vi "Send.vi"(8 "error in":errorcluster, 11 "Expedited Download Transfer in":refnum<class "Segmented Download Transfer.lvclass">) -> (0 "error out":errorcluster, 3 "Expedited Download Transfer out":refnum<class "Segmented Download Transfer.lvclass">)   [LabVIEW 2020, in "CANopen.lvlib" / "SDO Manager.lvlib" / "Segmented Download Transfer.lvclass"]
uses:
  Segmented Download Transfer.lvclass
  D:/git/CANopen-LabVIEW/source/SDO Manager/SDO Manager/SDO Transfer/SDO Transfer.lvclass
  SDO Transfer/SDO Transfer.lvclass/SDO Transfer.ctl
  CANopen Message/CANopen Message.lvclass/CANopen Message.ctl
  HAL/Source/Interfaces/ICommunicate/ICommunicate.lvclass
  CANopen Message/CANopen Message.lvclass
  Segmented Download Transfer.lvclass/Segmented Download Transfer.ctl
  Typedefs/Function Code.ctl
  CANopen.lvlib
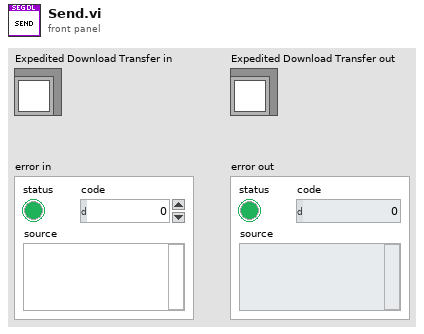
[diagram p1: front panel]
types:
  T1 = typedef "CANopen.lvlib/Function Code.ctl" = u8
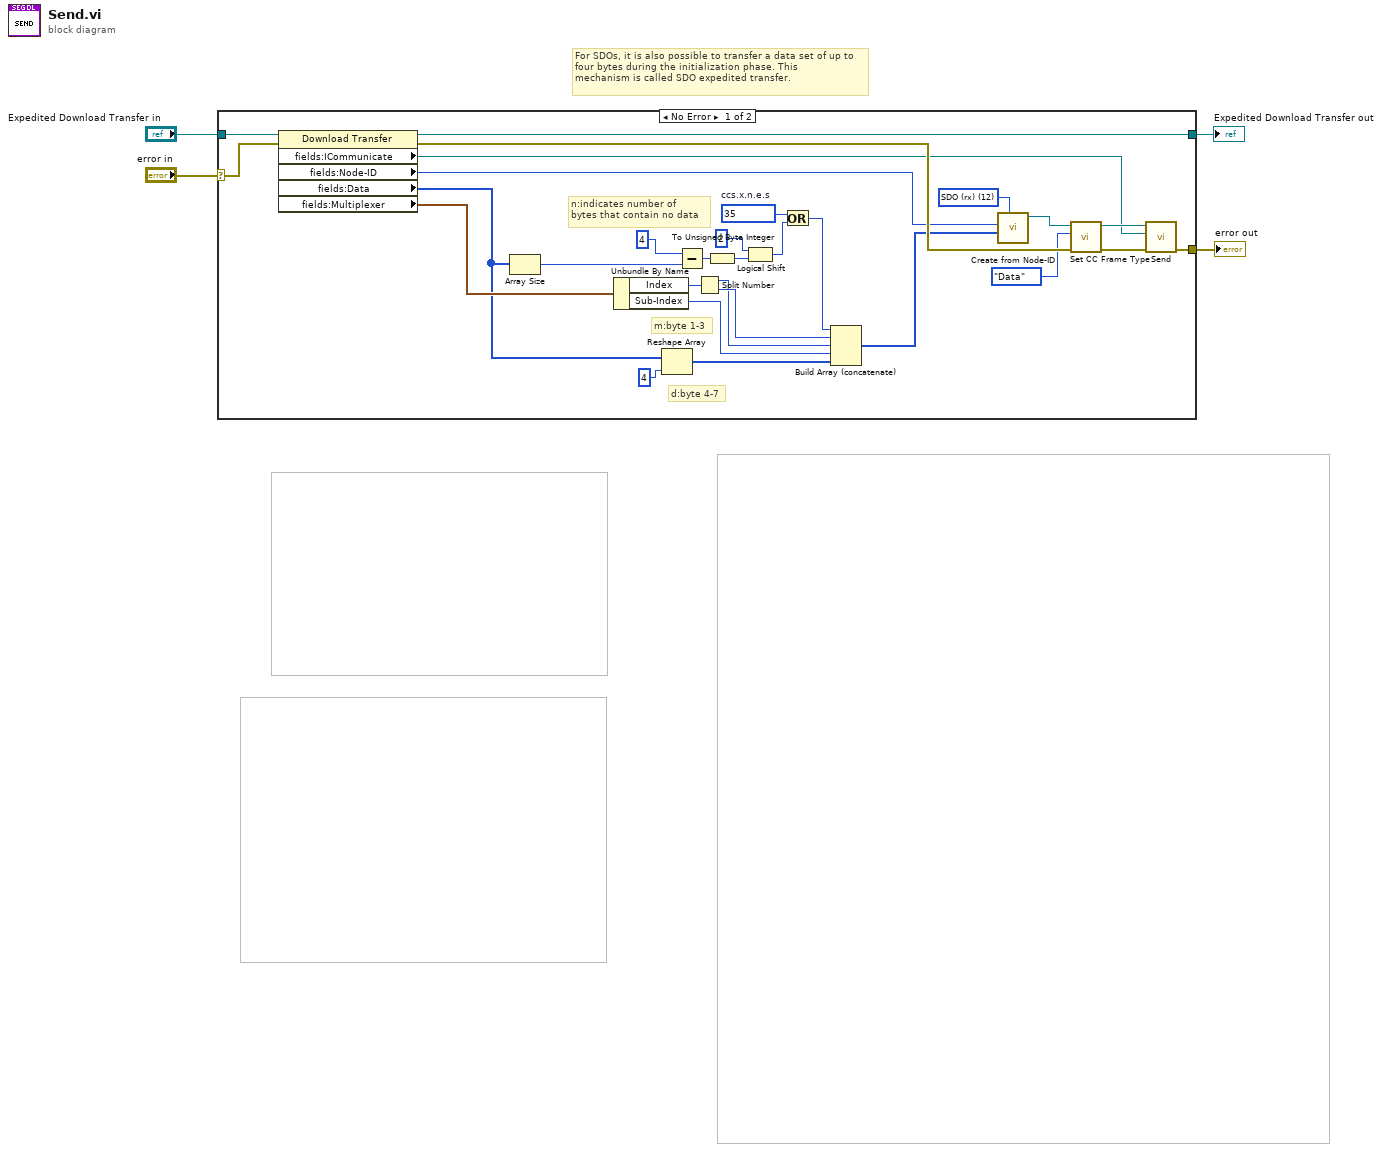
[diagram p0: block diagram]
diagram:
  # "For SDOs, it is also possible to transfer a data set of up to four bytes during the initialization phase. This \nmechanism is called SDO expedited transfer."
  n1 = case shown="No Error" "error in" {
    selector: "error in" -> [w32 w34]
    tunnel: "Expedited Download Transfer in" -> [w31 w35]
    tunnel: [w30 w35] -> w2
    tunnel: [w29 w34] -> w1
    frame No Error {
      w10 = T1 12 items=["NMT"=0, "EMCY/SYNC"=1, "TIME"=2, "PDO1 (tx)"=3, "PDO1 (rx)"=4, "PDO2 (tx)"=5, "PDO2 (rx)"=6, "PDO3 (tx)"=7, "PDO3 (rx)"=8, "PDO4 (tx)"=9, "PDO4 (rx)"=10, "SDO (tx)"=11, "SDO (rx)"=12, "NMT error control"=14] ("Function Code")
      w21 = u8 35  # ccs.x.n.e.s
      # "n:indicates number of\nbytes that contain no data"
      # "d:byte 4-7"
      # "m:byte 1-3"
      n2 = property class="Download Transfer"(reference=w31, error in=w32) -> (reference out=w30:refnum<class "Segmented Download Transfer.lvclass">, error out=w33:errorcluster, "fields:ICommunicate"=w5:refnum<class "ICommunicate.lvclass">, "fields:Node-ID"=w28:u8, "fields:Data"=w12:u8[], "fields:Multiplexer"=w14:cluster{"Index":u16, "Sub-Index":u8})
      n3 = Array Size(array=w12) -> (size(s)=w13:i32)
      n4 = Unbundle By Name(w14) -> ("Index"=w27:u16, "Sub-Index"=w24:u8)
      n5 = Reshape Array(w12, 4 ("y")) -> (w20:u8[])
      n6 = Subtract(x=4 ("y"), y=w13) -> (x-y=w18:i32)
      n7 = Split Number(x=w27) -> (hi(x)=w25:u8, lo(x)=w26:u8)
      n8 = To Unsigned Byte Integer(number=w18) -> (unsigned 8bit integer=w17:u8)
      n9 = Logical Shift(y=i8 2, x=w17) -> (x << y=w16:u8)
      n10 = Or(x=w21, y=w16) -> (x .or. y?=w22:u8)
      n11 = Build Array (concatenate)(w22, w26, w25, w24, w20) -> (w11:u8[])
      n12 = call "Create from Node-ID.vi"("Function Code"=w10, "Data"=w11, "Node-ID"=w28) -> ("CANopen Message"=w9:refnum<class "CANopen Message.lvclass">)  [unwired: 8 in]
      n13 = call "Set CC Frame Type.vi"("error in"=w33, "CC Frame Type"=enum8{"Data", "Remote", "Error", "Overload"}."Data", "CANopen Message in"=w9) -> ("error out"=w8:errorcluster, "CANopen Message out"=w7:refnum<class "CANopen Message.lvclass">)  [unwired: 7 in]
      n14 = call "Send.vi"("error in"=w8, "ICommunicate"=w5, "CANopen Message in"=w7) -> ("error out"=w29:errorcluster)  [unwired: 7 in, 1 out]
    }
    frame Error {
    }
  }
  "Expedited Download Transfer out" <- w2
  "error out" <- w1
